vi "UDMA_READ_FIFO.vi"(0 "TCP Network Connection in":refnum<k5>, 2 "N":u32=100, 5 "error in (no error)":errorcluster) -> (14 "TCP Network Connection out":refnum<k5>, 16 "Oscilloscope":u32[](graph), 18 "Status":u8[](array[numeric]), 19 "error out":errorcluster)   [LabVIEW 2019]
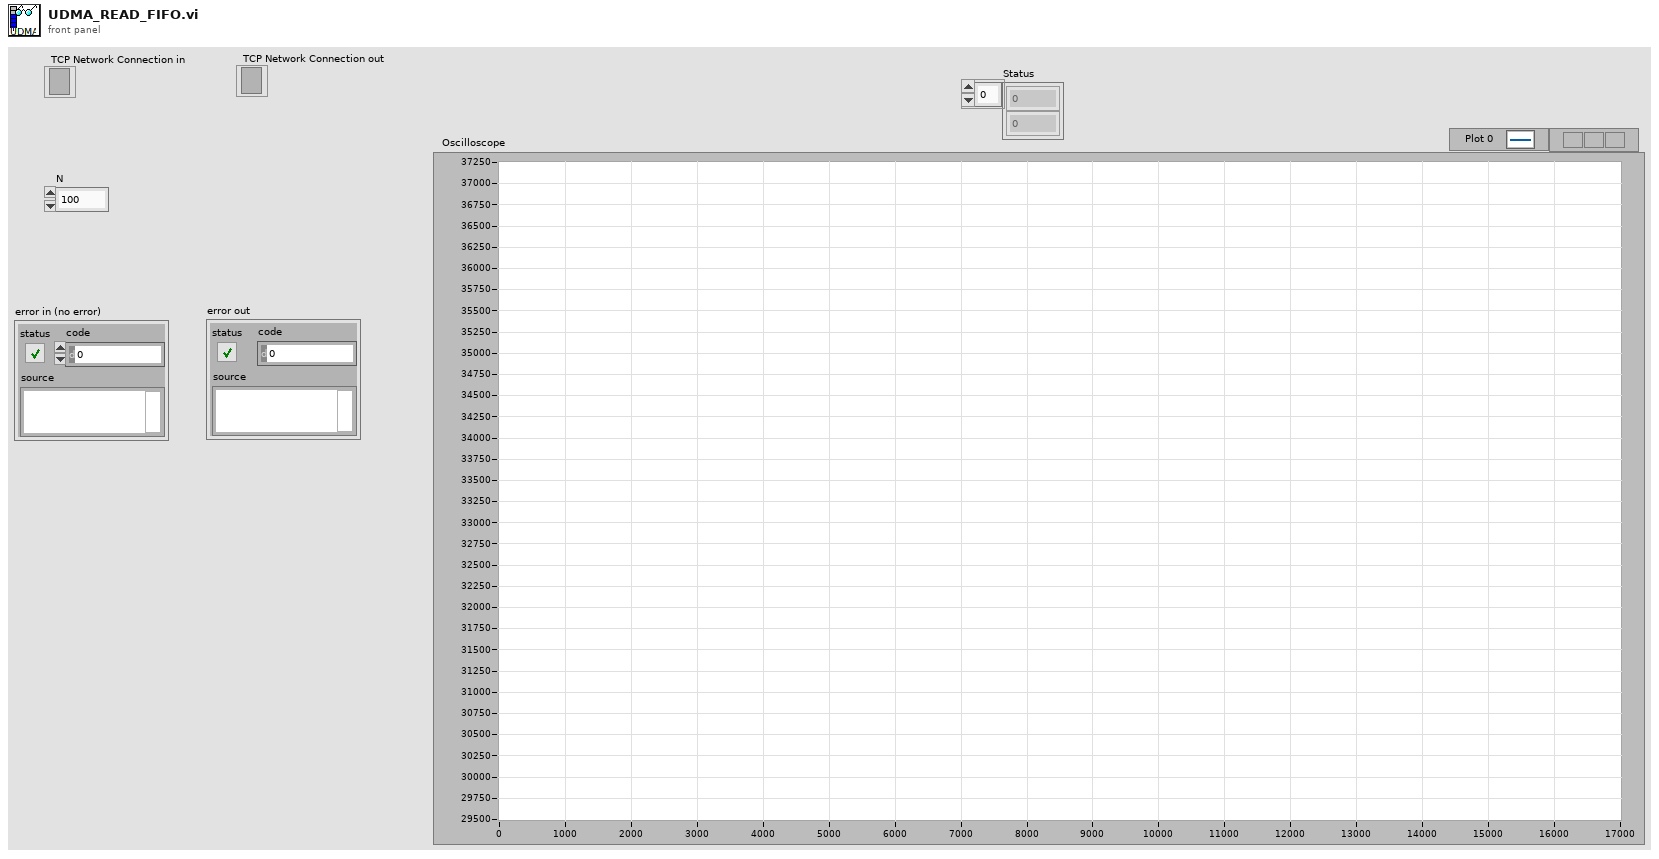
[diagram p1: front panel]
types:
  T1 = enum16{"big-endian, network order", "native, host order", "little-endian"}
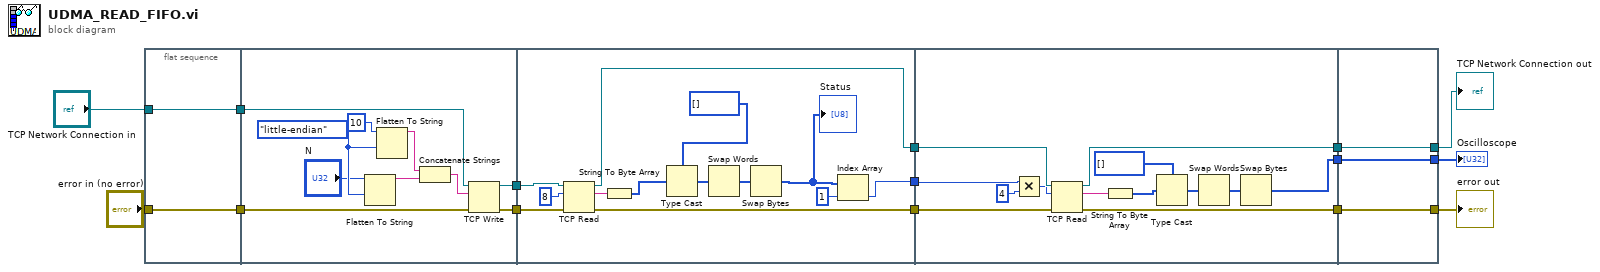
[diagram p0: block diagram]
diagram:
  n1 = flat-sequence {
    tunnel: [w16] -> w11
    tunnel: [w17] -> w10
    tunnel: "error in (no error)" -> [w17]
    tunnel: "TCP Network Connection in" -> [w16]
    tunnel: w11 -> [w27]
    tunnel: w10 -> [w26]
    tunnel: [w25] -> w5
    tunnel: [w24] -> w4
    tunnel: w5 -> [w37]
    tunnel: w4 -> [w40]
    tunnel: [w39] -> w3
    tunnel: [w29] -> w2
    tunnel: [w38] -> w1
    tunnel: w3 -> [w52]
    tunnel: w2 -> [w41]
    tunnel: [w51] -> w8
    tunnel: [w50] -> w7
    tunnel: [w42] -> w6
    tunnel: w1 -> [w53]
    tunnel: [w54] -> w9
    tunnel: [w55] -> w13
    tunnel: [w56] -> w12
    tunnel: w8 -> [w56]
    tunnel: w7 -> [w55]
    tunnel: w6 -> [w54]
    frame #0 {
    }
    frame #1 {
      w22 = T1."little-endian" ("byte order (0:big-endian, network order)")
      n2 = Flatten To String(anything="N", byte order (0:big-endian, network order)=w22) -> (data string=w23:string)  [unwired: 2 in, 2 out]
      n3 = Flatten To String(anything=u32 10 ("element"), byte order (0:big-endian, network order)=w22) -> (data string=w20:string)  [unwired: 2 in, 2 out]
      n4 = Concatenate Strings(w20, w23) -> (w19:string)
      n5 = TCP Write(connection ID=w27, data in=w19, error in (no error)=w26) -> (connection ID out=w25:refnum<k5>, error out=w24:errorcluster)  [unwired: 1 in, 1 out]
    }
    frame #2 {
      n6 = TCP Read(connection ID=w37, bytes to read=8, error in (no error)=w40) -> (connection ID out=w38:refnum<k5>, data out=w36:string, error out=w39:errorcluster)  [unwired: 2 in]
      n7 = String To Byte Array(string=w36) -> (unsigned byte array=w34:u8[])
      n8 = Type Cast(type=u32[] [], x=w34) -> (*(type *) &x=w33:u32[])
      n9 = Swap Words(1:w33) -> (0:w32:u32[])
      n10 = Swap Bytes(anything=w32) -> (byte swapped=w28:u32[])
      "Status" <- w28
      n11 = Index Array(array=w28, index=1) -> (element=w29:u32)
    }
    frame #3 {
      n12 = Multiply(x=w41, y=u32 4) -> (x*y=w49:u32)
      n13 = TCP Read(connection ID=w53, bytes to read=w49, error in (no error)=w52) -> (connection ID out=w51:refnum<k5>, data out=w43:string, error out=w50:errorcluster)  [unwired: 2 in]
      n14 = String To Byte Array(string=w43) -> (unsigned byte array=w47:u8[])
      n15 = Type Cast(type=u32[] [], x=w47) -> (*(type *) &x=w45:u32[])
      n16 = Swap Words(1:w45) -> (0:w44:u32[])
      n17 = Swap Bytes(anything=w44) -> (byte swapped=w42:u32[])
    }
    frame #4 {
    }
  }
  "error out" <- w13
  "TCP Network Connection out" <- w12
  "Oscilloscope" <- w9
